vi "Compute Target Distances.vi"(9 "Camera Type":enum16{"206", "1011", "1013"}(ring), 10 "Target Info":T4(array[cluster]), 11 "Image in":T3) -> (0 "Distances":T2(array[cluster]), 2 "Target Info":T5(array[cluster]), 3 "Image out":T3)   [LabVIEW 2013]
uses:
  Program Files/National Instruments/LabVIEW 2013/examples/FRC/Vision/2014 Target Detection/TargetType.ctl
  <vilib>/vision/Image Controls.llb/IMAQ Image.ctl
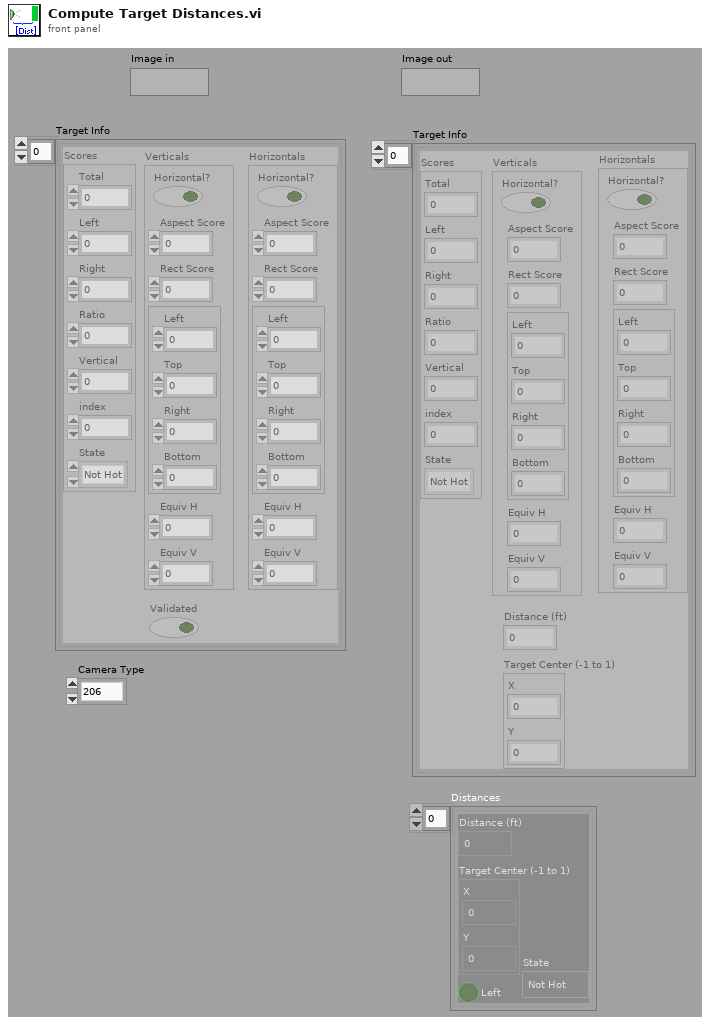
[diagram p1: front panel]
types:
  T1 = typedef "TargetType.ctl" = enum16{"Not Hot", "Hot"}
  T2 = cluster{"Distance (ft)":dbl, "Target Center (-1 to 1)":cluster{"X":dbl, "Y":dbl}, "Left":bool, "State":T1}[]
  T3 = typedef "IMAQ Image.ctl" = refnum<image>
  T4 = cluster{"Scores":cluster{"Total":dbl, "Left":dbl, "Right":dbl, "Ratio":dbl, "Vertical":dbl, "index":i32, "State":T1}, "Verticals":cluster{"Horizontal?":bool, "Aspect Score":dbl, "Rect Score":dbl, cluster{"Left":dbl, "Top":dbl, "Right":dbl, "Bottom":dbl}, "Equiv H":dbl, "Equiv V":dbl}, "Horizontals":cluster{"Horizontal?":bool, "Aspect Score":dbl, "Rect Score":dbl, cluster{"Left":dbl, "Top":dbl, "Right":dbl, "Bottom":dbl}, "Equiv H":dbl, "Equiv V":dbl}, "Validated":bool}[]
  T5 = cluster{"Scores":cluster{"Total":dbl, "Left":dbl, "Right":dbl, "Ratio":dbl, "Vertical":dbl, "index":i32, "State":T1}, "Verticals":cluster{"Horizontal?":bool, "Aspect Score":dbl, "Rect Score":dbl, cluster{"Left":dbl, "Top":dbl, "Right":dbl, "Bottom":dbl}, "Equiv H":dbl, "Equiv V":dbl}, "Horizontals":cluster{"Horizontal?":bool, "Aspect Score":dbl, "Rect Score":dbl, cluster{"Left":dbl, "Top":dbl, "Right":dbl, "Bottom":dbl}, "Equiv H":dbl, "Equiv V":dbl}, "Distance (ft)":dbl, "Target Center (-1 to 1)":cluster{"X":dbl, "Y":dbl}}[]
  T6 = cluster{"Total":dbl, "Left":dbl, "Right":dbl, "Ratio":dbl, "Vertical":dbl, "index":i32, "State":T1}
  T7 = cluster{"Horizontal?":bool, "Aspect Score":dbl, "Rect Score":dbl, cluster{"Left":dbl, "Top":dbl, "Right":dbl, "Bottom":dbl}, "Equiv H":dbl, "Equiv V":dbl}
  T8 = cluster{"Scores":cluster{"Total":dbl, "Left":dbl, "Right":dbl, "Ratio":dbl, "Vertical":dbl, "index":i32, "State":T1}, "Verticals":cluster{"Horizontal?":bool, "Aspect Score":dbl, "Rect Score":dbl, cluster{"Left":dbl, "Top":dbl, "Right":dbl, "Bottom":dbl}, "Equiv H":dbl, "Equiv V":dbl}, "Horizontals":cluster{"Horizontal?":bool, "Aspect Score":dbl, "Rect Score":dbl, cluster{"Left":dbl, "Top":dbl, "Right":dbl, "Bottom":dbl}, "Equiv H":dbl, "Equiv V":dbl}, "Distance (ft)":dbl, "Target Center (-1 to 1)":cluster{"X":dbl, "Y":dbl}}
  T9 = cluster{"Distance (ft)":dbl, "Target Center (-1 to 1)":cluster{"X":dbl, "Y":dbl}, bool, "State":T1}
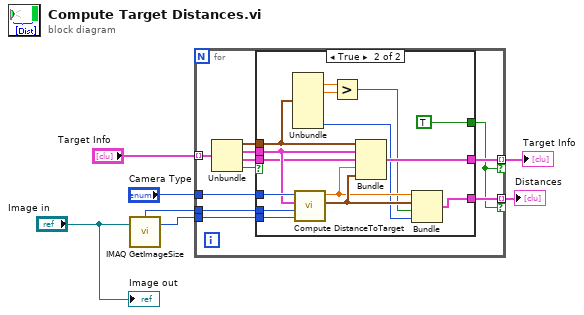
[diagram p0: block diagram]
diagram:
  n1 = call "IMAQ GetImageSize"("Image"="Image in") -> ("Y Resolution"=w6:i32, "X Resolution"=w5:i32)  [unwired: 3 in, 1 out]
  n2 = for {
    tunnel: "Target Info" -> [w18] mode=indexing
    tunnel: "Camera Type" -> [w15]
    tunnel: w5 -> [w14]
    tunnel: w6 -> [w13]
    tunnel: [w10] -> w7 mode=indexing if=w8
    tunnel: [w9] -> w1 mode=indexing if=w8
    n3 = Unbundle(w18) -> ("Scores"=w12:T6, "Verticals"=w16:T7, "Horizontals"=w11:T7, "Validated"=w17:bool)
    n4 = case shown="True" w17 {
      tunnel: w16 -> [_ w30]
      tunnel: w15 -> [_ w33]
      tunnel: w14 -> [_ w32]
      tunnel: w13 -> [_ w31]
      tunnel: w12 -> [_ w23]
      tunnel: w11 -> [_ w29]
      tunnel: [_ w28] -> w10
      tunnel: [_ TRUE] -> w8
      tunnel: [_ w24] -> w9
      frame False {
      }
      frame True {
        n5 = Unbundle(w23) -> ("Left"=w22:dbl, "Right"=w21:dbl, "State"=w19:T1)  [unwired: 4 out]
        n6 = call "Compute DistanceToTarget.vi"("Y Image Resolution"=w31, "X Image Resolution"=w32, "Vertical Strip"=w30, "Camera Type"=w33) -> ("Target Center (-1 to 1)"=w26:cluster{"X":dbl, "Y":dbl}, "Distance (ft)"=w25:dbl)  [unwired: 6 in]
        n7 = Greater?(x=w22, y=w21) -> (0:w20:bool)
        n8 = Bundle("Scores"=w23, "Verticals"=w30, "Horizontals"=w29, "Distance (ft)"=w25, "Target Center (-1 to 1)"=w26) -> (w28:T8)  [unwired: 1 in]
        n9 = Bundle("Distance (ft)"=w25, "Target Center (-1 to 1)"=w26, w20, "State"=w19) -> (w24:T9)  [unwired: 1 in]
      }
    }
  }
  "Target Info" <- w7
  "Distances" <- w1
  "Image out" <- "Image in"
